vi "Format String Constant.vi"(6 "Format String":string, 8 "error in":errorcluster, 11 "GObject in":refnum<vi>) -> (0 "error out":errorcluster, 2 "Successful":bool)   [LabVIEW 2019, in "Quick Format QD.lvlib"]
doc: "Formats a string constant based on the given Format String."
uses:
  Quick Format QD.lvlib
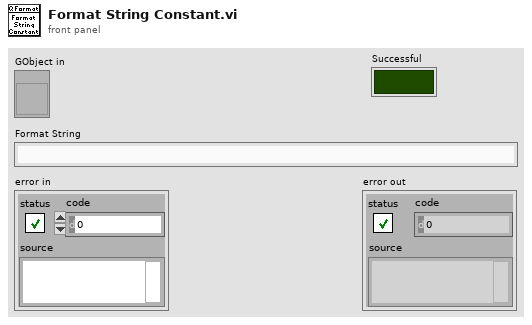
[diagram p1: front panel]
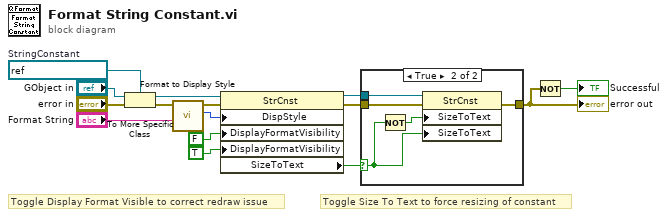
[diagram p0: block diagram]
diagram:
  w10 = refnum<vi> refnum  # StringConstant
  # "Toggle Size To Text to force resizing of constant"
  # "Toggle Display Format Visible to correct redraw issue"
  n1 = To More Specific Class(target class=w10, reference="GObject in", error in="error in") -> (specific class reference=w7:refnum<vi>, error out=w14:errorcluster)
  n2 = call "Format to Display Style.vi"("Format String"="Format String", "error in"=w14) -> ("Display Style"=w6:u32, "error out"=w13:errorcluster)  [unwired: 8 in]
  n3 = property on="Property Node" class="StrCnst"(reference=w7, error in=w13, "DispStyle"=w6, "DisplayFormatVisibility"=FALSE ("Display Format Visible?"), "DisplayFormatVisibility"=TRUE ("Display Format Visible?")) -> (reference out=w1:refnum<vi>, error out=w12:errorcluster, "SizeToText"=w2:bool)
  n4 = case shown="True" w2 {
    selector: w2 -> [_ w17]
    tunnel: w1 -> [_ w19]
    tunnel: w12 -> [w16 w21]
    tunnel: [w16 w20] -> w11
    frame False {
    }
    frame True {
      n5 = Not(x=w17) -> (.not. x?=w18:bool)
      n6 = property on="Property Node" class="StrCnst"(reference=w19, error in=w21, "SizeToText"=w18, "SizeToText"=w17) -> (error out=w20:errorcluster)  [unwired: 1 out]
    }
  }
  "error out" <- w11
  n7 = Not(x=w11) -> (.not. x?=→"Successful":bool)
